vi "Pass_List.vi"(8 "error in (no error)":errorcluster, 10 "Label.Text":string, 11 "Ref in":T1={"MS SQL Connection"=refnum, "UDL File"=path "", "Time"="", "DCODE"="", "WIP+1"=0, "MC No?"=0, "POKAYOKE?"=FALSE, "Expected Result"="", "Result [Status]"="", "Clock"=0.0, "RFID"="", "WIP Queue"=refnum, "TS Parameter"={"ProfitCenterCode"="", "LineCode"="", "WorkOrderNumber"="", "Model"="", "Model_with_Prefix"="", "VendorCode"="", "SetParameterDateCode"="", "PokaYoke"=0, "Target"=1, "Live_DateCode"="", "CustomerPartNumber"="", "Hand"="", "sBarcode"=FALSE, "FCA"=0, "Ent_Stamp"=timestamp(0 s since 1904-01-01), "STS_CD"=0.0}, "Data_Queue"=[], "RFID Serial No."=""} {"TS Parameter"."FCA" format="%01d"; "TS Parameter"."Target" min=1 max=100000; "TS Parameter"."PokaYoke" min=0 max=1}) -> (0 "error out":errorcluster)   [LabVIEW 2020]
uses:
  Controls/TD SQL.ctl
  <vilib>/addons/database/Connection.llb/Conn ObjectReference.ctl
  Controls/WIP_State.ctl
  Controls/TS_Parameter.ctl
  MS SQL/MS_Global.vi
  <vilib>/addons/database/NI_Database_API.lvlib
panel:
  in  "Exit":bool
  in  "WIP List":i32(listbox)
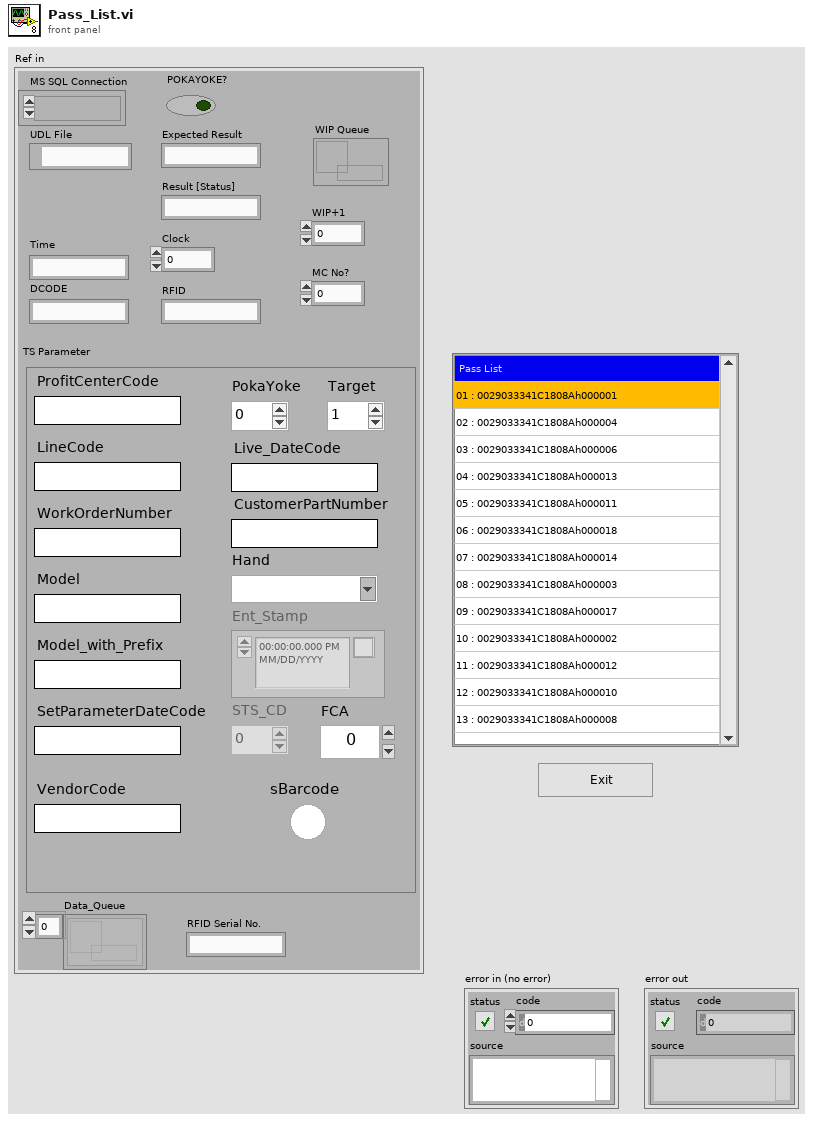
[diagram p1: front panel]
types:
  T1 = typedef "TD SQL.ctl" = cluster{"MS SQL Connection":T2, "UDL File":path, "Time":string, "DCODE":string, "WIP+1":i64, "MC No?":i32, "POKAYOKE?":bool, "Expected Result":string, "Result [Status]":string, "Clock":dbl, "RFID":string, "WIP Queue":refnum<queue>, "TS Parameter":T3, "Data_Queue":refnum<queue>[], "RFID Serial No.":string}
  T2 = typedef "NI_Database_API.lvlib/Conn ObjectReference.ctl" = refnum<k1>
  T3 = typedef "TS_Parameter.ctl" = cluster{"ProfitCenterCode":string, "LineCode":string, "WorkOrderNumber":string, "Model":string, "Model_with_Prefix":string, "VendorCode":string, "SetParameterDateCode":string, "PokaYoke":i32, "Target":i32, "Live_DateCode":string, "CustomerPartNumber":string, "Hand":string, "sBarcode":bool, "FCA":i32, "Ent_Stamp":timestamp, "STS_CD":dbl}
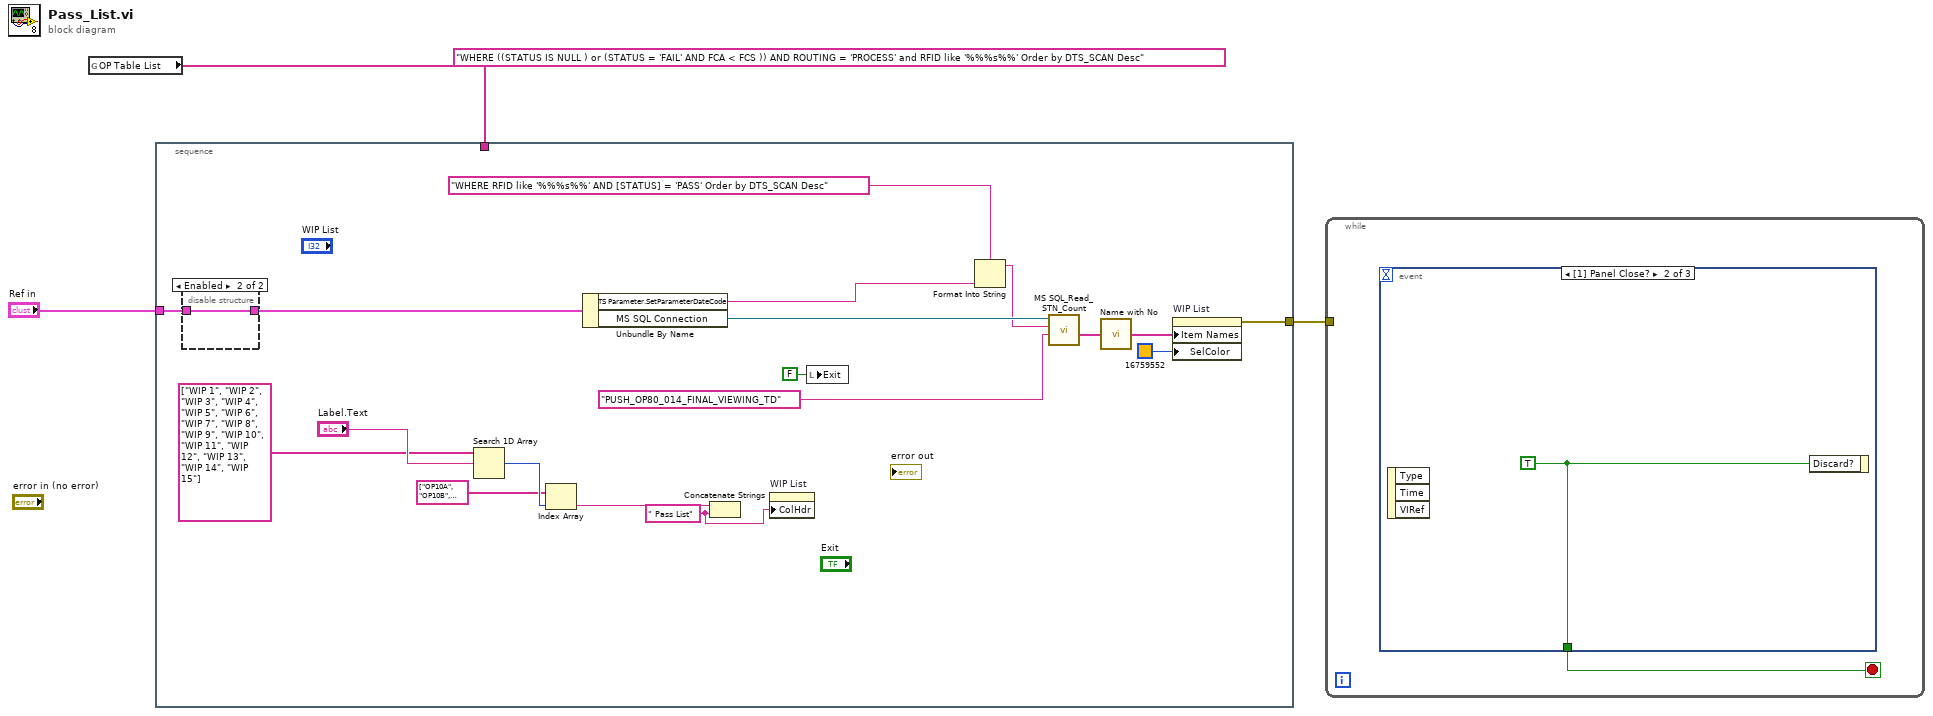
[diagram p0: block diagram]
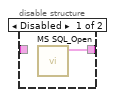
[diagram p2: hidden frame]
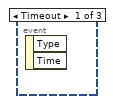
[diagram p3: hidden frame]
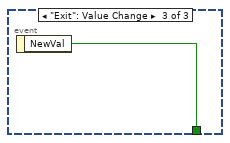
[diagram p4: hidden frame]
diagram:
  (unwired) "WHERE ((STATUS IS NULL ) or (STATUS = 'FAIL' AND FCA < FCS )) AND ROUTING = 'PROCESS' and RFID like '%%%s%%' Order by DTS_SCAN Desc" ("Query")
  n1 = global read "MS_Global.vi" "OP Table List"() -> (w2:string[])
  n2 = stacked-sequence {
    tunnel: [w15] -> w3
    tunnel: w2 -> [_]
    tunnel: "Ref in" -> [w6]
    frame #0 {
      w8 = " Pass List" ("string")
      n3 = disable-structure shown="Enabled" {
        disable-tunnel: w6 -> [_ w23]
        disable-tunnel: [w22 w23] -> w5
        frame Disabled {
          n4 = call "MS SQL_Open.vi"() -> ("Ref Out"=w22:T1)  [unwired: 9 in, 2 out]
        }
        frame Enabled {
        }
      }
      n5 = Search 1D Array(1D array=string[] ["WIP 1", "WIP 2", "WIP 3", "WIP 4", "WIP 5", "WIP 6", "WIP 7", "WIP 8", "WIP 9", "WIP 10", "WIP 11", "WIP 12", "WIP 13", "WIP 14", "WIP 15"], element="Label.Text") -> (index of element=w11:i32)  [unwired: 1 in]
      n6 = Index Array(array=string[] ["OP10A", "OP10B", "OP20A", "OP20B", "OP30A", "OP30B", "OP30C", "OP40A", "OP40B", "OP50A", "OP50B", "OP60", "OP70", "OP80"] ("Array"), index=w11) -> (element=w9:string)
      n7 = Unbundle By Name(w5) -> ("TS Parameter.SetParameterDateCode"=w4:string, "MS SQL Connection"=w19:T2)
      n8 = Concatenate Strings(w9, w8) -> ()  [unwired: 1 out]
      n9 = property on="WIP List" class="LstBox (strict)"("ColHdr"=w8) -> ()  [unwired: 2 in, 2 out]
      n10 = local write "Exit"(FALSE ("Exit")) -> ()
      n11 = Format Into String(format string="WHERE RFID like '%%%s%%' AND [STATUS] = 'PASS' Order by DTS_SCAN Desc" ("Query"), w4) -> (resulting string=w17:string)  [unwired: 2 in, 1 out]
      n12 = call "MS SQL_Read_STN_Count.vi"("Table?"="PUSH_OP80_014_FINAL_VIEWING_TD" ("Label.Text"), "Query"=w17, "Refnum in"=w19) -> ("RFID"=w13:string[])  [unwired: 5 in, 3 out]
      n13 = call <userlib>:"Name with No.vi"("Seq Name In"=w13) -> ("Seq Name (No.)"=w16:string[])  [unwired: 14 in]
      n14 = property on="WIP List" class="LstBox (strict)"("Item Names"=w16, "SelColor"=u32 16759552 ("Selection Color")) -> (error out=w15:errorcluster)  [unwired: 2 in, 1 out]
    }
  }
  n15 = while {
    tunnel: w3 -> [_]
    stop <- w24 stop-if-true
    n16 = event shown="[1] Panel Close?" {
      selector: _ -> [_ _ _]
      dyn-events: _ -> [_ _ _]
      timeout: _ -> [_ _ _]
      tunnel: [_ w25 w26] -> w24
      event Timeout {
        n17 = event-data() -> ()  [unwired: 1 in, 2 out]
      }
      event Panel Close? {
        w25 = TRUE ("Discard?")
        n18 = event-data() -> ()  [unwired: 1 in, 3 out]
        n19 = event-data("Discard?"=w25) -> ()  [unwired: 1 in, 1 out]
      }
      event "Exit": Value Change {
        n20 = event-data() -> ("NewVal"=w26:bool)  [unwired: 1 in]
      }
    }
  }
